vi "Refresh from Plots Config.vi"(8 "error in (no error)":errorcluster, 11 "HistorianCharting in":refnum<class "HistorianCharting.lvclass">) -> (0 "error out":errorcluster, 3 "HistorianCharting out":refnum<class "HistorianCharting.lvclass">)   [LabVIEW 2020, in "VolatusGUIElements.lvlib" / "HistorianCharting.lvclass"]
uses:
  HistorianCharting.lvclass
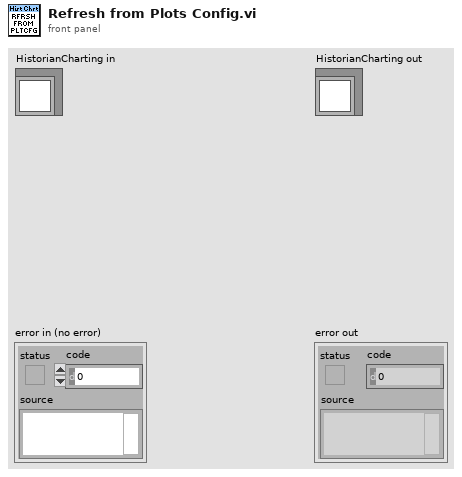
[diagram p1: front panel]
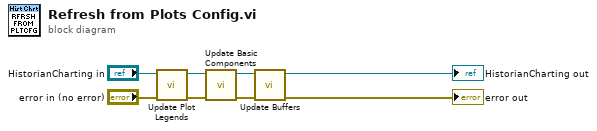
[diagram p0: block diagram]
diagram:
  n1 = call "Update Plot Legends.vi"("error in (no error)"="error in (no error)", "HistorianCharting in"="HistorianCharting in") -> ("error out"=w7:errorcluster, "HistorianCharting out"=w5:refnum<class "HistorianCharting.lvclass">)  [unwired: 8 in]
  n2 = call "Update Basic Components.vi"("error in (no error)"=w7, "HistorianCharting in"=w5) -> ("error out"=w4:errorcluster, "HistorianCharting out"=w2:refnum<class "HistorianCharting.lvclass">)  [unwired: 8 in]
  n3 = call "Update Buffers.vi"("error in (no error)"=w4, "HistorianCharting in"=w2) -> ("error out"=→"error out":errorcluster, "HistorianCharting out"=→"HistorianCharting out":refnum<class "HistorianCharting.lvclass">)  [unwired: 8 in]
